vi "Init AnalogIn.vi"(7 "ADC #":T1=-1, 8 "error in (no error)":errorcluster, 11 "VisaSession in":refnum<class "VisaComms.lvclass">) -> (0 "error out":errorcluster, 2 "AnalogIn":refnum<class "AI.lvclass">, 3 "VisaSession out":refnum<class "VisaComms.lvclass">)   [LabVIEW 2020]
uses:
  VisaComms.lvclass/VisaComms.ctl
  AI/AI.lvclass
  Session/Session.lvclass
  VisaComms.lvclass
  ADC Number.ctl
  CTI.lvlib
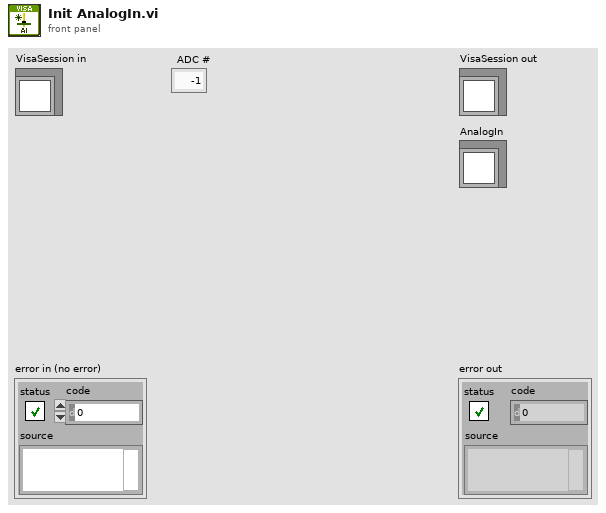
[diagram p1: front panel]
types:
  T1 = typedef "CTI.lvlib/ADC Number.ctl" = i8
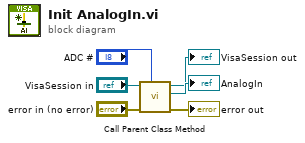
[diagram p0: block diagram]
diagram:
  n1 = call-parent "Call Parent Class Method"(7:"ADC #", "error in (no error)"="error in (no error)", "Session in"="VisaSession in") -> ("error out"=→"error out":errorcluster, "AnalogIn"=→"AnalogIn":refnum<class "AnalogIn.lvclass">, "Session out"=→"VisaSession out":refnum<class "Session.lvclass">)  [unwired: 6 in]
